vi "通讯.vi"() -> ()   [LabVIEW 2016, in "流量计集成.lvlib" / "LDM51明渠流量计.lvlib"]
uses:
  <vilib>/Analysis/baseanly.llb/Mean (DBL).vi
  <vilib>/Plasmionique/MB Master/MB_Master_Serial/MB_Master_Serial.lvclass
  C:/Program Files (x86)/National Instruments/LabVIEW 2016/vi.lib/Plasmionique/MB Master/MB_Master/MB_Master.lvclass
  <vilib>/Plasmionique/MB Master/MB Master.lvlib
  <vilib>/Analysis/NI_AALBase.lvlib
panel:
  out "总累积流量":dbl
  out "总流量":dbl
  out "平均流速":dbl
  out "平均水位":dbl
  out "累积流量":u32[](array[numeric])
  out "流速":dbl[](array[numeric])
  out "流量":dbl[](array[numeric])
  out "水位":dbl[](array[numeric])
  out "流量计启用":bool[](array[boolean])
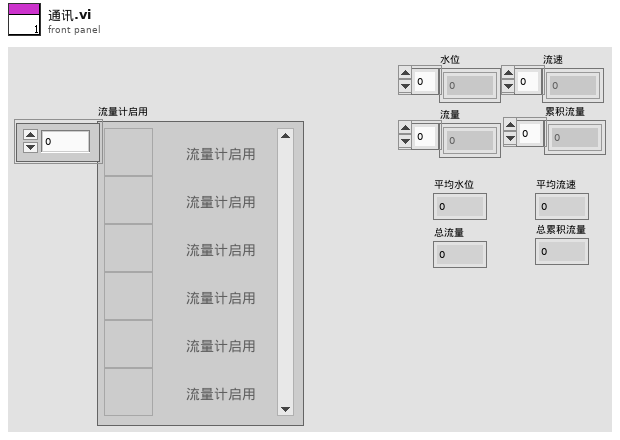
[diagram p1: front panel]
types:
  T1 = cluster{"baud rate (bps)":u32, "stop bits":u16, "parity":u16, "flow control":u16, "timeout":u32, "retries":i32}
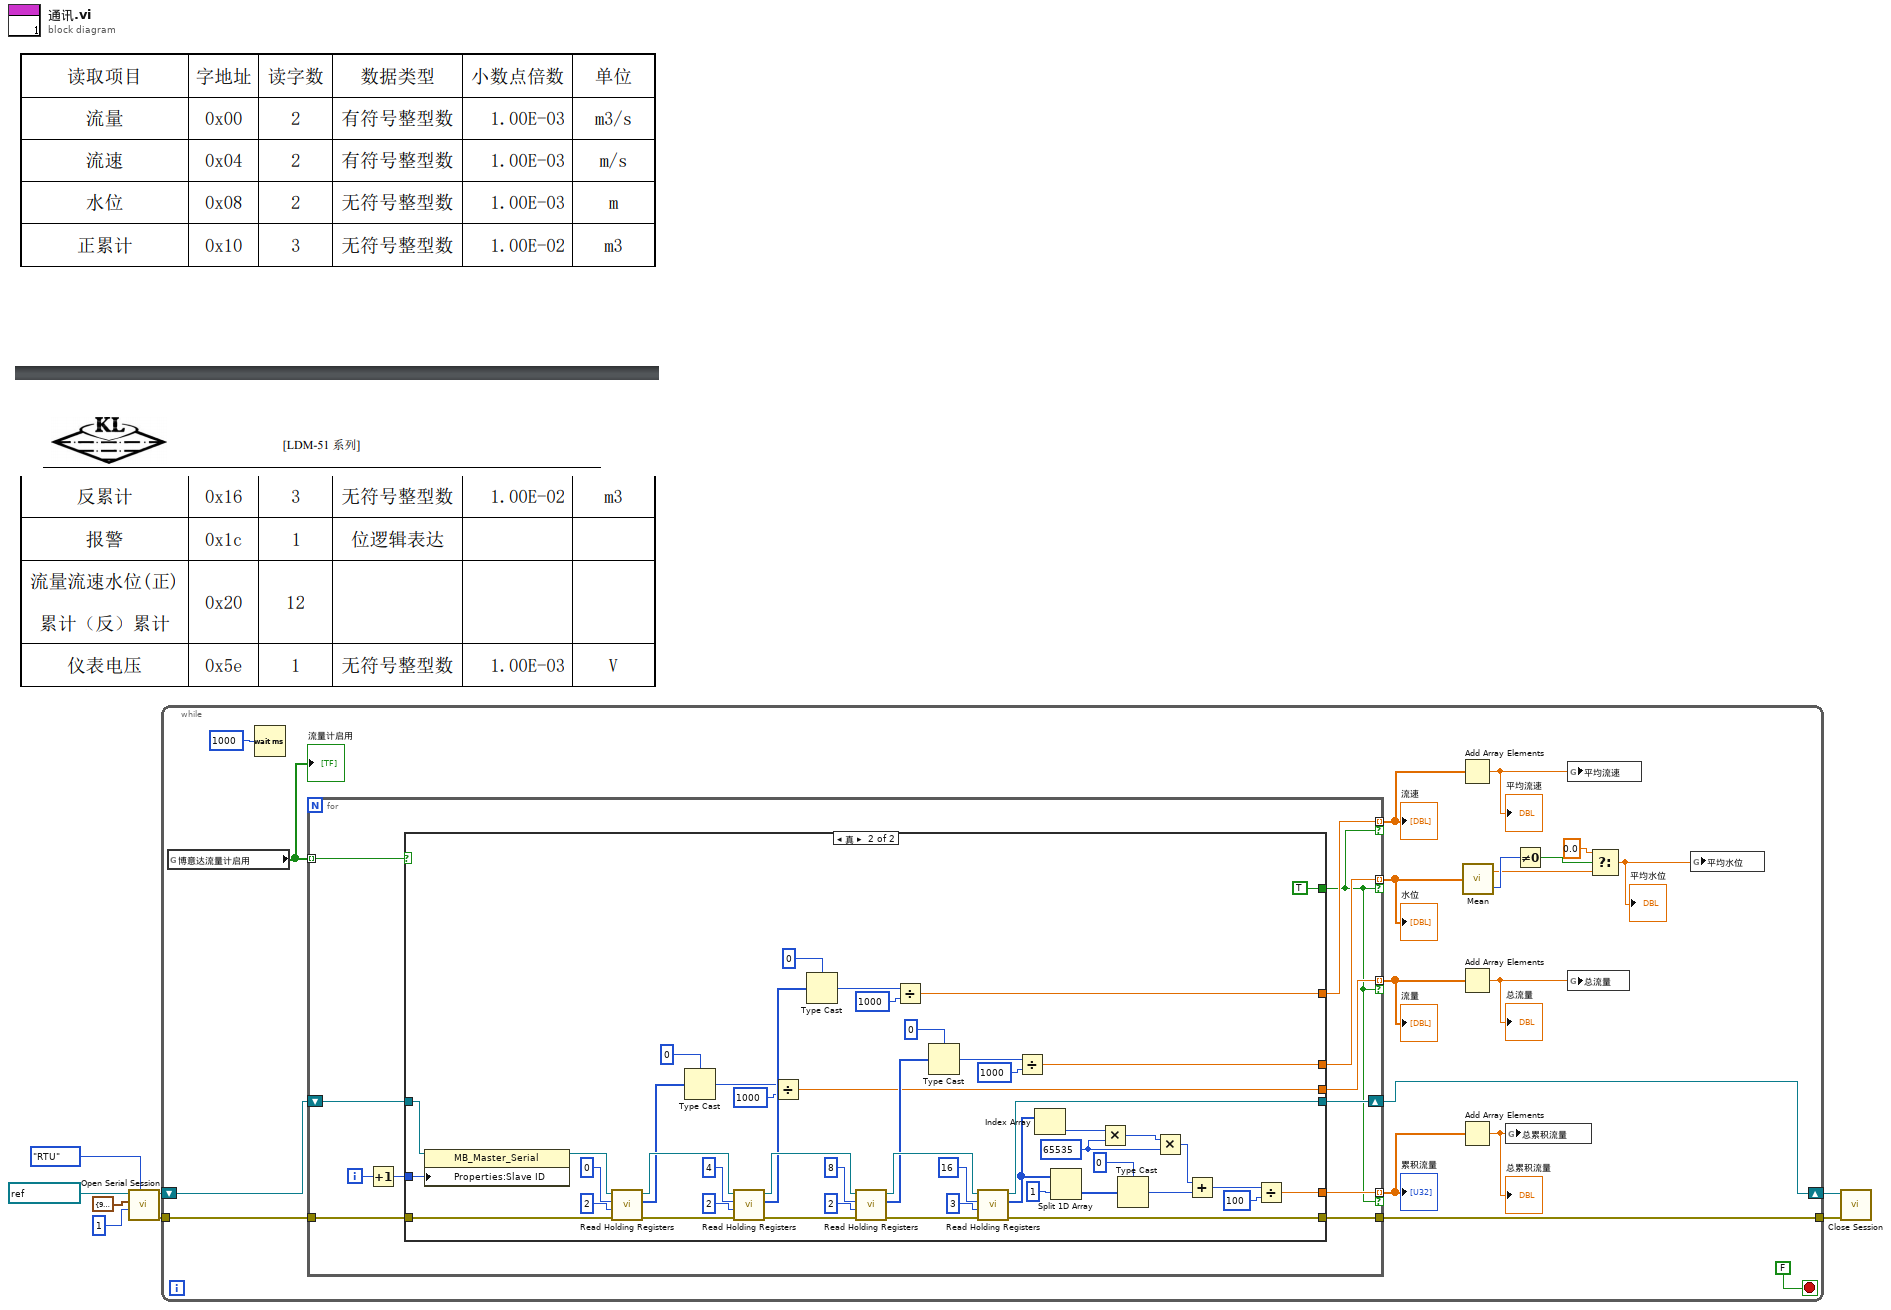
[diagram p0: block diagram]
diagram:
  n1 = call <vilib>:"Open Serial Session.vi"("Mode (RTU)"=enum16{"RTU", "ASCII"}."RTU", "Slave ID"=u8 1, "Serial Config"=T1 {"baud rate (bps)"=9600, "stop bits"=10, "parity"=0, "flow control"=0, "timeout"=1000, "retries"=1}, "VISA Resource"=refnum<visa-resource-name> "COM10") -> ("Error out"=w6:errorcluster, "MB_Serial session"=w1:refnum<class "MB_Master_Serial.lvclass">)  [unwired: 6 in]
  n2 = while {
    tunnel: w6 -> [w27]
    shift-right: [w26] -> w8
    shift-left: w1 -> [w22]
    tunnel: [w25] -> w7
    stop <- FALSE stop-if-true
    n3 = global read "流量计全局变量.vi" "博意达流量计启用"() -> (w16:bool[])
    "流量计启用" <- w16
    n4 = Wait (ms)(milliseconds to wait=u32 1000 ("等待时间（毫秒）")) -> ()  [unwired: 1 out]
    n5 = for {
      shift-right: [w38] -> w26
      shift-left: w22 -> [w36]
      tunnel: w16 -> [w33] mode=indexing
      tunnel: [w32] -> w19 mode=indexing if=w28
      tunnel: [w31] -> w21 mode=indexing if=w28
      tunnel: [w30] -> w20 mode=indexing if=w28
      tunnel: [w29] -> w15 mode=indexing if=w28
      tunnel: w27 -> [w39]
      tunnel: [w37] -> w25
      i -> [w35]
      n6 = Increment(x=w35) -> (x+1=w34:i32)
      n7 = case shown="真" w33 {
        tunnel: w39 -> [w40 w89]
        tunnel: [w41 w75] -> w38
        tunnel: [w40 w74] -> w37
        tunnel: w36 -> [w41 w63]
        tunnel: w34 -> [_ w61]
        tunnel: [_ w60] -> w32
        tunnel: [_ w59] -> w31
        tunnel: [_ w42] -> w30
        tunnel: [_ w58] -> w29
        tunnel: [_ TRUE] -> w28
        frame False {
        }
        frame True {
          w46 = u32 65535 ("y")
          n8 = property class="MB_Master_Serial"(reference=w63, "Properties:Slave ID"=w61) -> (reference out=w62:refnum<class "MB_Master_Serial.lvclass">)  [unwired: 1 in, 1 out]
          n9 = call <vilib>:"Read Holding Registers.vi"("error in (no error)"=w89, "quantity"=u16 2, "starting address"=u16 0, "MB session in"=w62) -> ("error out"=w85:errorcluster, "Registers"=w73:u16[], "MB session out"=w86:refnum<class "MB_Master_Serial.lvclass">)  [unwired: 5 in]
          n10 = Type Cast(type=0, x=w73) -> (*(type *) &x=w57:i32)
          n11 = call <vilib>:"Read Holding Registers.vi"("error in (no error)"=w85, "quantity"=u16 2, "starting address"=u16 4, "MB session in"=w86) -> ("error out"=w79:errorcluster, "Registers"=w72:u16[], "MB session out"=w82:refnum<class "MB_Master_Serial.lvclass">)  [unwired: 5 in]
          n12 = Divide(x=w57, y=1000) -> (x/y=w60:dbl)
          n13 = Type Cast(type=0, x=w72) -> (*(type *) &x=w55:i32)
          n14 = call <vilib>:"Read Holding Registers.vi"("error in (no error)"=w79, "quantity"=u16 2, "starting address"=u16 8, "MB session in"=w82) -> ("error out"=w77:errorcluster, "Registers"=w70:u16[], "MB session out"=w78:refnum<class "MB_Master_Serial.lvclass">)  [unwired: 5 in]
          n15 = Divide(x=w55, y=1000) -> (x/y=w58:dbl)
          n16 = Type Cast(type=0, x=w70) -> (*(type *) &x=w56:i32)
          n17 = call <vilib>:"Read Holding Registers.vi"("error in (no error)"=w77, "quantity"=u16 3, "starting address"=u16 16, "MB session in"=w78) -> ("error out"=w74:errorcluster, "Registers"=w53:u16[], "MB session out"=w75:refnum<class "MB_Master_Serial.lvclass">)  [unwired: 5 in]
          n18 = Divide(x=w56, y=1000) -> (x/y=w59:dbl)
          n19 = Index Array(array=w53) -> (element=w48:u16)  [unwired: 1 in]
          n20 = Split 1D Array(array=w53, index=1 ("索引")) -> (second subarray=w51:u16[])  [unwired: 1 out]
          n21 = Multiply(x=w48, y=w46) -> (x*y=w47:u32)
          n22 = Type Cast(type=0, x=w51) -> (*(type *) &x=w49:i32)
          n23 = Multiply(x=w47, y=w46) -> (x*y=w45:u32)
          n24 = Add(x=w45, y=w49) -> (x+y=w44:u32)
          n25 = Divide(x=w44, y=100) -> (x/y=w42:dbl)
        }
      }
    }
    "水位" <- w21
    "流量" <- w19
    "流速" <- w15
    "累积流量" <- w20
    n26 = Add Array Elements(numeric array=w15) -> (sum=w14:dbl)
    "平均流速" <- w14
    n27 = Add Array Elements(numeric array=w19) -> (sum=w17:dbl)
    "总流量" <- w17
    n28 = Add Array Elements(numeric array=w20) -> (sum=w18:dbl)
    "总累积流量" <- w18
    n29 = call-poly <vilib>:"Mean.vi"("X"=w21) -> ("mean"=w10:dbl, "error"=w13:i32)
    n30 = global write "流量计全局变量.vi" "总累积流量"(w18) -> ()
    n31 = Not Equal To 0?(x=w13) -> (x != 0?=w12:bool)
    n32 = global write "流量计全局变量.vi" "平均流速"(w14) -> ()
    n33 = global write "流量计全局变量.vi" "总流量"(w17) -> ()
    n34 = Select(t=0.0, s=w12, f=w10) -> (s? t:f=w9:dbl)
    "平均水位" <- w9
    n35 = global write "流量计全局变量.vi" "平均水位"(w9) -> ()
  }
  n36 = call-dynamic "Close Session.vi"("error in (no error)"=w7, "MB_Serial session"=w8) -> ()  [unwired: 9 in, 1 out]
